vi "Init.vi"(8 "error in (no error)":errorcluster, 11 "DAQmx Digitizer in":refnum<class "DAQmx Digitizer.lvclass">) -> (0 "error out":errorcluster, 3 "DAQmx Digitizer out":refnum<class "DAQmx Digitizer.lvclass">)   [LabVIEW 2015, in "DAQmx Digitizer.lvclass"]
uses:
  DAQmx Digitizer.lvclass
  DAQmx Digitizer.lvclass/DAQmx Digitizer.ctl
  <vilib>/DAQmx/create/channels.llb/DAQmx Create Channel (AI-Voltage-Basic).vi
  <vilib>/DAQmx/configure/timing.llb/DAQmx Timing (Sample Clock).vi
  <vilib>/DAQmx/configure/trigger.llb/DAQmx Reference Trigger (Digital Edge).vi
  <resource>/objmgr/daqmx.rc
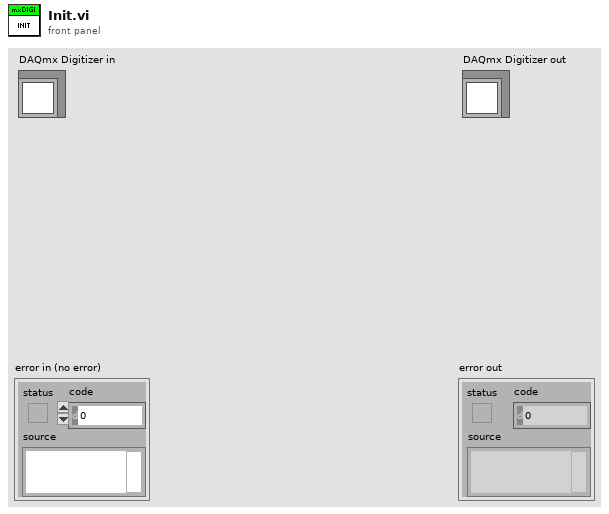
[diagram p1: front panel]
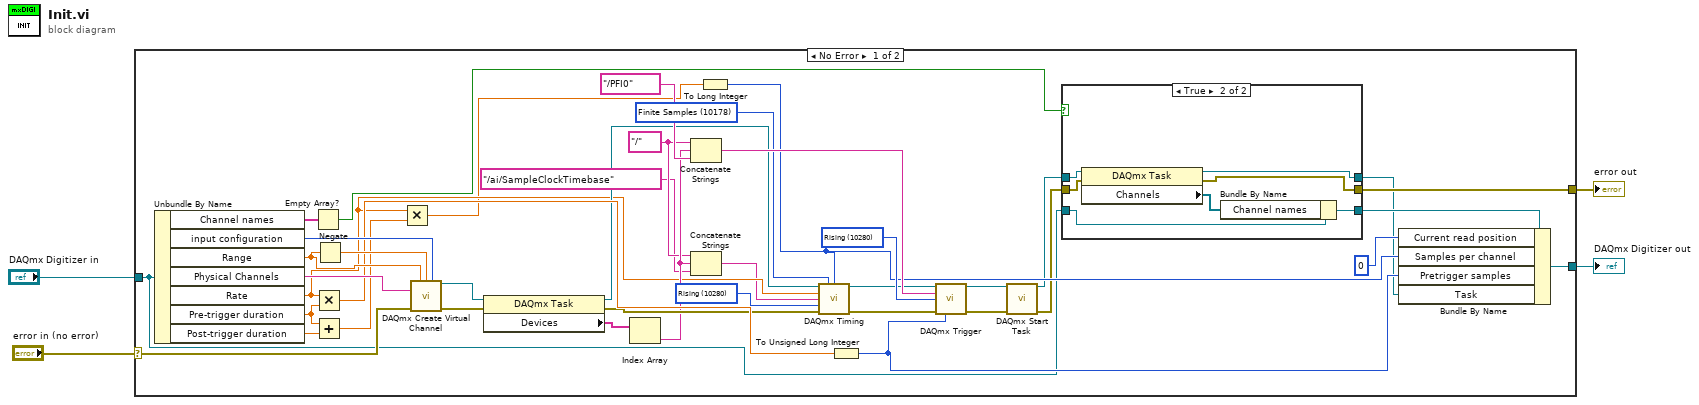
[diagram p0: block diagram]
diagram:
  n1 = case shown="No Error" "error in (no error)" {
    selector: "error in (no error)" -> [w44 w57]
    tunnel: [w10 w57] -> w3
    tunnel: [w35 w56] -> w1
    tunnel: "DAQmx Digitizer in" -> [w7 w56]
    frame No Error {
      w15 = 10280 items=["Rising"=10280, "Falling"=10171] ("active edge")
      w22 = 10178 items=["Finite Samples"=10178, "Continuous Samples"=10123, "Hardware Timed Single Point"=12522] ("sample mode")
      w24 = tag "/" ("string")
      w37 = 10280 items=["Rising"=10280, "Falling"=10171] ("edge")
      n2 = Unbundle By Name(w7) -> ("Channel names"=w9:string[], "input configuration"=w39:i32, "Range"=w43:dbl, "Physical Channels"=w45:tag, "Rate"=w18:dbl, "Pre-trigger duration"=w21:dbl, "Post-trigger duration"=w20:dbl)
      n3 = Empty Array?(array=w9) -> (empty?=w8:bool)
      n4 = Multiply(x=w18, y=w21) -> (x*y=w34:dbl)
      n5 = Add(x=w21, y=w20) -> (x+y=w19:dbl)
      n6 = Negate(x=w43) -> (-x=w42:dbl)
      n7 = Multiply(x=w18, y=w19) -> (x*y=w17:dbl)
      n8 = call-poly <vilib>:"DAQmx Create Virtual Channel.vi"("maximum value"=w43, "minimum value"=w42, "input terminal configuration"=w39, "physical channels"=w45, "error in"=w44) -> ("task out"=w41:refnum<k21>, "error out"=w36:errorcluster)  [unwired: 9 in]
      n9 = property class="DAQmx Task"(reference=w41, error in=w36) -> (reference out=w29:refnum<k21>, error out=w28:errorcluster, "Devices"=w40:tag[])
      n10 = Index Array(array=w40) -> (element=w25:tag)  [unwired: 1 in]
      n11 = Concatenate Strings(w24, w25, tag "/PFI0" ("string")) -> (w30:string)
      n12 = Concatenate Strings(w24, w25, tag "/ai/SampleClockTimebase" ("string")) -> (w14:string)
      n13 = To Long Integer(number=w17) -> (32bit integer=w16:i32)
      n14 = call-poly <vilib>:"DAQmx Timing.vi"("task/channels in"=w29, "sample mode"=w22, "samples per channel"=w16, "rate"=w18, "source"=w14, "active edge"=w15, "error in"=w28) -> ("task out"=w26:refnum<k21>, "error out"=w27:errorcluster)  [unwired: 7 out]
      n15 = To Unsigned Long Integer(number=w34) -> (unsigned 32bit integer=w33:u32)
      n16 = call-poly <vilib>:"DAQmx Trigger.vi"("task/channels in"=w26, "source"=w30, "edge"=w37, "error in"=w27, "pretrigger samples per channel"=w33) -> ("task out"=w31:refnum<k21>, "error out"=w32:errorcluster)  [unwired: 9 out]
      n17 = call <vilib>:"DAQmx Start Task.vi"("task/channels in"=w31, "error in"=w32) -> ("task out"=w12:refnum<k21>, "error out"=w11:errorcluster)  [unwired: 12 out]
      n18 = case shown="True" w8 {
        tunnel: w12 -> [w46 w55]
        tunnel: w11 -> [w48 w54]
        tunnel: [w48 w53] -> w10
        tunnel: w7 -> [w47 w52]
        tunnel: [w47 w50] -> w6
        tunnel: [w46 w49] -> w5
        frame False {
        }
        frame True {
          n19 = property class="DAQmx Task"(reference=w55, error in=w54) -> (reference out=w49:refnum<k21>, error out=w53:errorcluster, "Channels"=w51:refnum<k21>[])
          n20 = Bundle By Name(cluster=w52, "Channel names"=w51) -> (w50:refnum<class "DAQmx Digitizer.lvclass">)
        }
      }
      n21 = Bundle By Name(cluster=w6, "Current read position"=0, "Samples per channel"=w16, "Pretrigger samples"=w33, "Task"=w5) -> (w35:refnum<class "DAQmx Digitizer.lvclass">)
    }
    frame Error {
    }
  }
  "error out" <- w3
  "DAQmx Digitizer out" <- w1
